vi "PH_Switch_USB.ProcEvents.vi"(0 "i ref in":refnum<vi>, 5 "error in (no error)":errorcluster) -> (14 "i ref out":refnum<vi>, 19 "error out":errorcluster)   [LabVIEW 2014, in "PH_Switch_USB.lvlib"]
doc: "This method is used to define the events the object will listen to. Add your own events here."
uses:
  PH_Switch_USB.lvlib
  CS_Core/BaseProcess/BaseProcess.event definition.ctl
  CS_Core/CAEObj/CAEObj.event definition.ctl
  CS_Core/BaseProcess/BaseProcess.descriptor string definition.ctl
  CS_Core/BaseProcess/BaseProcess.lvlib
  CS_Core/CAEObj/CAEObj.lvlib
  PH_Basics/PH_Common/PH_Common.lvlib
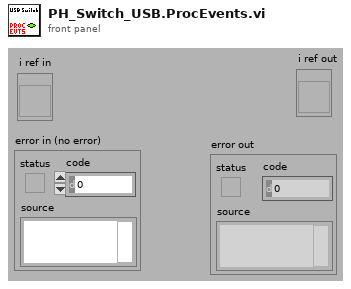
[diagram p1: front panel]
types:
  T1 = typedef "BaseProcess.lvlib/BaseProcess.event definition.ctl" = cluster{"CAEEvtDef":T2, "Data Descriptor":T3}
  T2 = typedef "CAEObj.lvlib/CAEObj.event definition.ctl" = cluster{"URL":string, "enable":bool, "ignoreResID":bool}
  T3 = typedef "BaseProcess.lvlib/BaseProcess.descriptor string definition.ctl" = string
  T4 = typedef "PH_Switch_USB.lvlib/PH_Switch_USB.i attribute.ctl" = cluster{"GUI Refs":cluster{"GUI-Knob":refnum<vi>, "Delete":refnum<vi>}, "Switch":cluster{"GUI Ref":refnum<vi>, "Service name":string, "Array No.":i16, "caption":string, "Status":T5}, "True-Sensor":cluster{"GUI Ref":refnum<vi>, "Service name":string, "Array No.":i16, "caption":string, "Status":T5}, "False-Sensor":cluster{"GUI Ref":refnum<vi>, "Service name":string, "Array No.":i16, "caption":string, "Status":T5}}
  T5 = typedef "PH_StatusHandler.lvlib/PH_StatusHandler.Status.ctl" = i16
  T6 = typedef "PH_Common.lvlib/PH_DIM.Event Declarer.ctl" = cluster{"Service Name":string, "Selector":string}
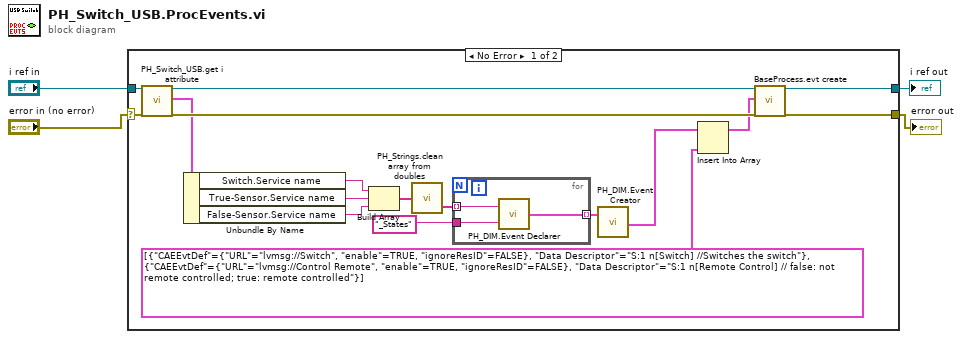
[diagram p0: block diagram]
diagram:
  n1 = case shown="No Error" "error in (no error)" {
    selector: "error in (no error)" -> [w5 w25]
    tunnel: "i ref in" -> [w14 w26]
    tunnel: [w13 w26] -> w3
    tunnel: [w12 w25] -> w2
    frame No Error {
      n2 = call "PH_Switch_USB.get i attribute.vi"("i ref in"=w14, "error in (no error)"=w5) -> ("i ref out"=w21:refnum<vi>, "i attribute"=w19:T4, "error out"=w20:errorcluster)  [unwired: 15 in]
      n3 = Unbundle By Name(w19) -> ("Switch.Service name"=w18:string, "True-Sensor.Service name"=w17:string, "False-Sensor.Service name"=w16:string)
      n4 = Build Array(w18, w17, w16) -> (w11:string[])
      n5 = call "PH_Strings.clean array from doubles.vi"("Array Input"=w11) -> ("Cleaned Array Output"=w9:string[])  [unwired: 1 out]
      n6 = for {
        tunnel: [w22] -> w10 mode=indexing
        tunnel: w9 -> [w24] mode=indexing
        tunnel: "_States" -> [w23]
        n7 = call "PH_DIM.Event Declarer.vi"("Selector"=w23, "Service Name"=w24) -> ("declared DIM Event"=w22:T6)
      }
      n8 = call "PH_DIM.Event Creator.vi"("Trendmessage Services"=w10) -> ("DIM Service Events"=w7:T1[])  [unwired: 18 in]
      n9 = Insert Into Array(array=w7, new element=T1[] [{"CAEEvtDef"={"URL"="lvmsg://Switch", "enable"=TRUE, "ignoreResID"=FALSE}, "Data Descriptor"="S:1 n[Switch] //Switches the switch"}, {"CAEEvtDef"={"URL"="lvmsg://Control Remote", "enable"=TRUE, "ignoreResID"=FALSE}, "Data Descriptor"="S:1 n[Remote Control] // false: not remote controlled; true: remote controlled"}] ("new events")) -> (w15:T1[])  [unwired: 1 in]
      n10 = call "BaseProcess.evt create.vi"("i ref in"=w21, "newEvents"=w15, "error in (no error)"=w20) -> ("i ref out"=w13:refnum<vi>, "error out"=w12:errorcluster)  [unwired: 13 in, 2 out]
    }
    frame Error {
    }
  }
  "i ref out" <- w3
  "error out" <- w2
